vi "WPI_SolenoidSetBool.vi"(8 "error in (no error)":errorcluster, 10 "Value":bool, 11 "SolenoidDevRef":T1={"DevStatus"={"status"=FALSE, "code"=0, "source"=""}, "Pneumatics Control Module"=0, "Forward Solenoid Channel"=enum."Invalid", "Reverse Solenoid Channel"=enum."Invalid"}) -> (0 "error out":errorcluster, 3 "SolenoidDevRef":T1={"DevStatus"={"status"=FALSE, "code"=0, "source"=""}, "Pneumatics Control Module"=0, "Forward Solenoid Channel"=enum."Invalid", "Reverse Solenoid Channel"=enum."Invalid"})   [LabVIEW 2017]
doc: "Specifies whether the NI 9472 sends a 12 V signal to the solenoid you specify. When the solenoid receives the 12 V signal, the solenoid releases air, thus moving the associated robot part.\n\nThis software is licensed. Open the labview\\readme\\WPI Robotics Library Open Source License.txt file for more information."
uses:
  <vilib>/Rock Robotics/WPI/Solenoid/WPI_SolenoidDevRef.ctl
  <vilib>/Rock Robotics/WPI/Solenoid/WPI_SolenoidChannel.ctl
  <vilib>/Rock Robotics/WPI/Solenoid/WPI_SolenoidCacheOp.ctl
  <vilib>/Rock Robotics/WPI/CAN/PCM/WPI_CAN_PCMGlobalOps.ctl
  <vilib>/Rock Robotics/WPI/Solenoid/WPI_SolenoidSafetyCheck.vi
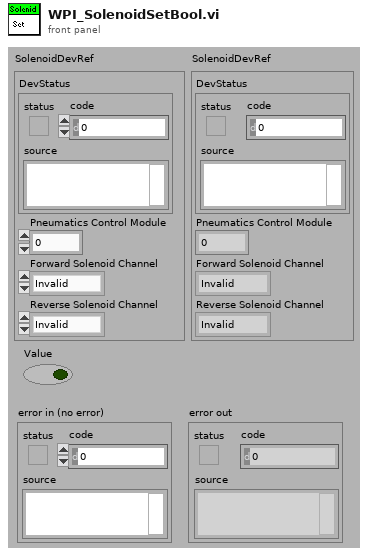
[diagram p1: front panel]
types:
  T1 = typedef "WPI_SolenoidDevRef.ctl" = cluster{"DevStatus":errorcluster, "Pneumatics Control Module":u8, "Forward Solenoid Channel":T2, "Reverse Solenoid Channel":T2}
  T2 = typedef "WPI_SolenoidChannel.ctl" = enum8{"Solenoid 0", "Solenoid 1", "Solenoid 2", "Solenoid 3", "Solenoid 4", "Solenoid 5", "Solenoid 6", "Solenoid 7", "Invalid"}
  T3 = typedef "WPI_SolenoidCacheOp.ctl" = enum16{"Acquire", "Release", "Status"}
  T4 = typedef "WPI_CAN_PCMGlobalOps.ctl" = enum16{"Read For Send", "Write After Receive", "Set Solenoids", "Set Closed Loop", "Clear Sticky Faults", "Get All", "Write Error", "Write After Receive Blacklist", "Set Control Frame Rate"}
  T5 = cluster{"Solenoid Status":bool[], "Battery Voltage":dbl, "Solenoid Voltage":dbl, "Compressor Current":dbl, "CompressorEnabled":bool, "StickySolenoidFault":bool, "StickyCompressorFault":bool, "SolenoidFault":bool, "CompressorFault":bool, "HardwareFault":bool, "ClosedLoopStatus":bool, "PressureStatus":bool, "Module Enabled":bool, "ClosedLoopSuggestedOutput":bool, "CAN Error":errorcluster, "Sticky Solenoid Faults":bool[]}
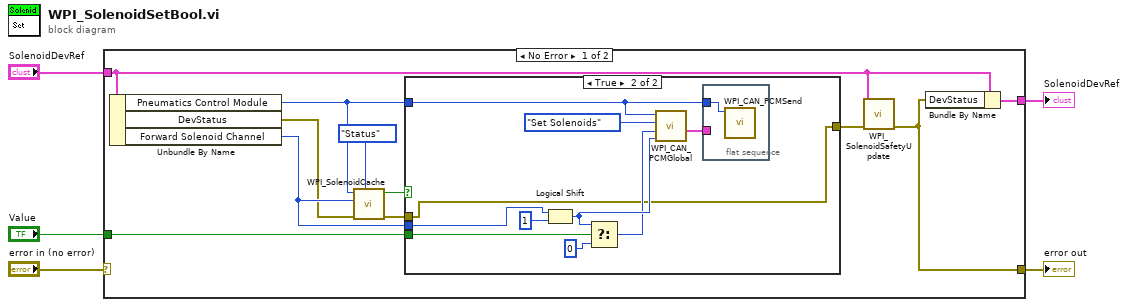
[diagram p0: block diagram]
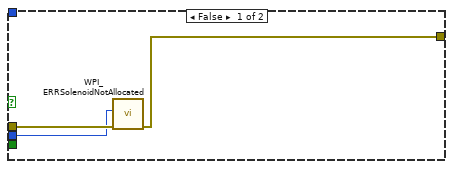
[diagram p2: hidden frame]
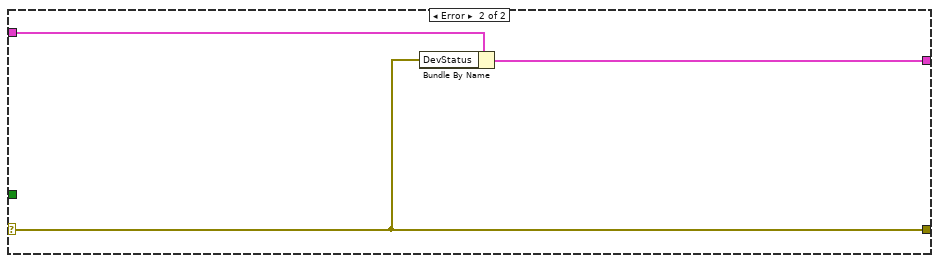
[diagram p3: hidden frame]
diagram:
  n1 = case shown="No Error" "error in (no error)" {
    selector: "error in (no error)" -> [_ w31]
    tunnel: "SolenoidDevRef" -> [w6 w33]
    tunnel: "Value" -> [w16 _]
    tunnel: [w7 w31] -> w2
    tunnel: [w15 w32] -> w1
    frame No Error {
      n2 = Unbundle By Name(w6) -> ("Pneumatics Control Module"=w14:u8, "DevStatus"=w12:errorcluster, "Forward Solenoid Channel"=w13:T2)
      n3 = call <vilib>:"WPI_SolenoidCache.vi"("AllocatedSolenoidOp"=WPI_SolenoidCacheOp."Status", "error in (no error)"=w12, "SolenoidChannel"=w13, "Pneumatics Control Module"=w14) -> ("error out"=w10:errorcluster, "Allocated"=w11:bool)  [unwired: 6 out]
      n4 = case shown="True" w11 {
        tunnel: w16 -> [_ w26]
        tunnel: [w19 w22] -> w8
        tunnel: w14 -> [_ w21]
        tunnel: w13 -> [w17 w28]
        tunnel: w10 -> [w18 w22]
        frame False {
          n5 = call <vilib>:"WPI_ERRSolenoidNotAllocated.vi"("error in (no error)"=w18, "Solenoid Channel"=w17) -> ("error out"=w19:errorcluster)  [unwired: 9 in]
        }
        frame True {
          n6 = Logical Shift(y=w28, x=u8 1) -> (x << y=w25:u8)
          n7 = Select(t=w25, s=w26, f=u8 0) -> (s? t:f=w24:u8)
          n8 = call <vilib>:"WPI_CAN_PCMGlobal.vi"("Solenoid Set Mask"=w25, "Solenoid Set Value"=w24, "Operation"=WPI_CAN_PCMGlobalOps."Set Solenoids", "Pneumatics Control Module (0)"=w21) -> ("Get All"=w20:T5)  [unwired: 5 in, 2 out]
          n9 = flat-sequence {
            tunnel: w21 -> [w30]
            tunnel: w20 -> [_]
            frame #0 {
              n10 = call <vilib>:"WPI_CAN_PCMSend.vi"("Pneumatics Control Module (0)"=w30) -> ()  [unwired: 10 in, 1 out]
            }
          }
        }
      }
      n11 = call <vilib>:"WPI_SolenoidSafetyUpdate.vi"("error in (no error)"=w8, "SolenoidDevRef"=w6) -> ("error out"=w7:errorcluster)  [unwired: 9 out]
      n12 = Bundle By Name(cluster=w6, "DevStatus"=w7) -> (w15:T1)
    }
    frame Error {
      n13 = Bundle By Name(cluster=w33, "DevStatus"=w31) -> (w32:T1)
    }
  }
  "SolenoidDevRef" <- w1
  "error out" <- w2
